vi "Write SA Pin.vi"(8 "error in (no error)":errorcluster, 10 "SA Pin":string, 11 "PAE in":refnum<class "PAE.lvclass">=refnum) -> (0 "error out":errorcluster, 3 "PAE out":refnum<class "PAE.lvclass">)   [LabVIEW 2016, in "SeqAuto Evaluations.lvlib" / "PAE.lvclass"]
uses:
  PAE.lvclass
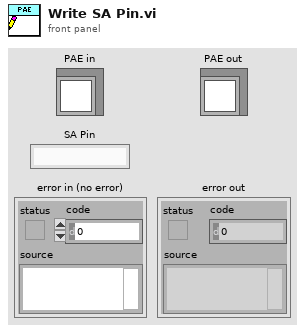
[diagram p1: front panel]
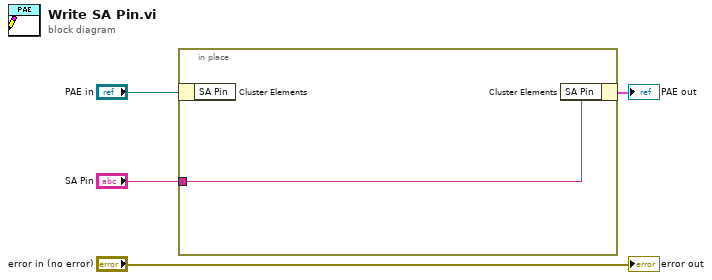
[diagram p0: block diagram]
diagram:
  n1 = in-place {
    in-place-border: "SA Pin" -> [w5]
    n2 = in-place-cluster #1("PAE in") -> ()  [unwired: 1 out]
    n3 = in-place-cluster #1("SA Pin"=w5) -> (→"PAE out":cluster{})
  }
  "error out" <- "error in (no error)"
